vi "Windows.Exit.vi"(7 "Exit Action":T1=enum."Log off PC user") -> (0 "error out":errorcluster)   [LabVIEW 2019, in "Tools.lvlib"]
doc: "This VI allows you to exit windows in various ways.\nexit windows function\n0: Log off\n1: Shut Down\n2: Exit Windows and reboot the computer"
uses:
  Tools.lvlib
  Windows.ExitAction.ctl
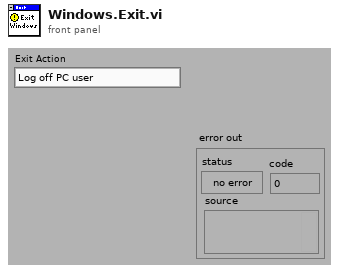
[diagram p1: front panel]
types:
  T1 = typedef "Tools.lvlib/Windows.ExitAction.ctl" = enum16{"Close TMOS", "Log off PC user", "Shut down the computer", "Reboot the computer"}
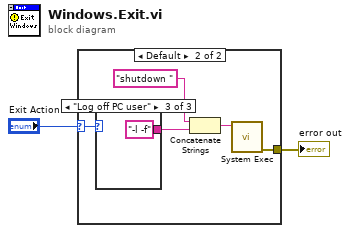
[diagram p0: block diagram]
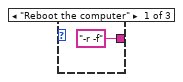
[diagram p3: hidden frame]
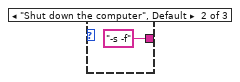
[diagram p4: hidden frame]
diagram:
  n1 = case shown="Default" "Exit Action" {
    selector: "Exit Action" -> [_ w7]
    tunnel: [_ w6] -> w2
    frame "Close TMOS" {
    }
    frame Default {
      n2 = case shown="\"Log off PC user\"" w7 {
        tunnel: ["-r -f" "-s -f" "-l -f"] -> w3
        frame "Reboot the computer" {
        }
        frame "Shut down the computer", Default {
        }
        frame "Log off PC user" {
        }
      }
      n3 = Concatenate Strings("shutdown " ("command line"), w3) -> (w4:string)
      n4 = call <vilib>:"System Exec.vi"("command line"=w4) -> ("error out"=w6:errorcluster)  [unwired: 7 in, 3 out]
    }
  }
  "error out" <- w2
